vi "Finish.vi"   [LabVIEW 2012]
doc: "This VI is called just before exiting. It is expected to close I/O refnum, save collected data, etc."
uses:
  <vilib>/Rock Robotics/WPI/Compressor/WPI_CompressorGetSetRefNum.vi
  <vilib>/Rock Robotics/WPI/Joystick/WPI_JoystickGetSetRefNum.vi
  <vilib>/Rock Robotics/WPI/RobotDrive/WPI_RobotDriveGetSetRefNum.vi
types:
  T1 = typedef "WPI_EncoderDevRef.ctl" = cluster{"DevStatus":errorcluster, "EncoderIndex":T2, "CounterIndex":T3, "DistancePerCount":dbl, "Decoding Type":T4}
  T2 = typedef "FPGA_EncoderIdx.ctl" = enum8{"Enc 0", "Enc 1", "Enc 2", "Enc 3", "Invalid"}
  T3 = typedef "FPGA_CounterCtrSystemIndex.ctl" = enum8{"Ctr 0", "Ctr 1", "Ctr 2", "Ctr 3", "Ctr 4", "Ctr 5", "Ctr 6", "Ctr 7", "Invalid"}
  T4 = typedef "WPI_EncoderType.ctl" = enum16{"1x", "2x", "4x"}
  T5 = typedef "WPI_CompressorDevRef.ctl" = cluster{"DevStatus":errorcluster, "DigitalInputDevRef":T6, "RelayDevRef":T9}
  T6 = typedef "WPI_DigitalInputDevRef.ctl" = cluster{"DevStatus":errorcluster, "DIO Channel":T7, "Digital Module":T8}
  T7 = typedef "FPGA_DIOChannel.ctl" = enum8{"DIO 1", "DIO 2", "DIO 3", "DIO 4", "DIO 5", "DIO 6", "DIO 7", "DIO 8", "DIO 9", "DIO 10", "DIO 11", "DIO 12", "DIO 13", "DIO 14", "Invalid"}
  T8 = typedef "FPGA_TypedefDigitalModule.ctl" = enum16{"Digital Module 1", "Digital Module 2"}
  T9 = typedef "WPI_RelayDevRef.ctl" = cluster{"DevStatus":errorcluster, "Relay Channel":T10, "Digital Module":T8, "Relay Direction":T11}
  T10 = typedef "FPGA_DIORelayChannel.ctl" = enum8{"Relay 1", "Relay 2", "Relay 3", "Relay 4", "Relay 5", "Relay 6", "Relay 7", "Relay 8", "Invalid"}
  T11 = typedef "WPI_RelayDirection.ctl" = enum16{"Both directions", "Forward only", "Reverse only"}
  T12 = typedef "WPI_SolenoidDevRef.ctl" = cluster{"DevStatus":errorcluster, "Solenoid Module":T13, "Forward Solenoid Channel":T14, "Reverse Solenoid Channel":T14}
  T13 = typedef "FPGA_TypedefSolenoidModule.ctl" = enum16{"Solenoid Module 1", "Solenoid Module 2"}
  T14 = typedef "WPI_SolenoidChannel.ctl" = enum8{"Solenoid 1", "Solenoid 2", "Solenoid 3", "Solenoid 4", "Solenoid 5", "Solenoid 6", "Solenoid 7", "Solenoid 8", "Invalid"}
  T15 = typedef "WPI_CameraDevRef.ctl" = cluster{"Camera Address":string, "CameraStatus":errorcluster, "Acquire Image Notifier":refnum<notifier>}
  T16 = typedef "WPI_JoystickDevRef.ctl" = cluster{"Device":T17}
  T17 = typedef "WPI_JoystickDeviceEnum.ctl" = enum16{"USB 1", "USB 2", "USB 3", "USB 4", "Kinect 1", "Kinect 2"}
  T18 = typedef "WPI_RobotDriveDevRef.ctl" = cluster{"DevStatus":errorcluster, "Motors[]":T19[], "Square Inputs":bool, "Max Output":dbl, "Isochronous":bool}
  T19 = typedef "WPI_MotorControlDeviceRef.ctl" = cluster{"DeviceStatus":errorcluster, "Type":enum16{"PWM", "CAN"}, "PWM":cluster{"Digital Module":T8, "PWM Channel":T20, "DeadBand":T21}, "CAN":cluster{"Device Number":u8, "Control Mode":T22, "Semaphore":T23, "Max Vout":dbl}, "Invert":bool, "TransformRef":T24, "InvTransformRef":T24}
  T20 = typedef "FPGA_DIOPWMChannel.ctl" = enum8{"PWM 1", "PWM 2", "PWM 3", "PWM 4", "PWM 5", "PWM 6", "PWM 7", "PWM 8", "PWM 9", "PWM 10", "Invalid"}
  T21 = typedef "WPI_PWMDeadband.ctl" = cluster{"Name":string, "maxPositivePwm":i32, "minPositivePwm":i32, "centerPwm":i32, "maxNegativePwm":i32, "minNegativePwm":i32, "angularRange":u16}
  T22 = typedef "WPI_CANJaguar_ControlMode.ctl" = enum8{"Percent VBus", "Current", "Speed", "Position", "Voltage"}
  T23 = typedef "Semaphore RefNum" = refnum<k1>
  T24 = typedef "WPI_PWMTransform_ConPane.ctl" = refnum<vi>
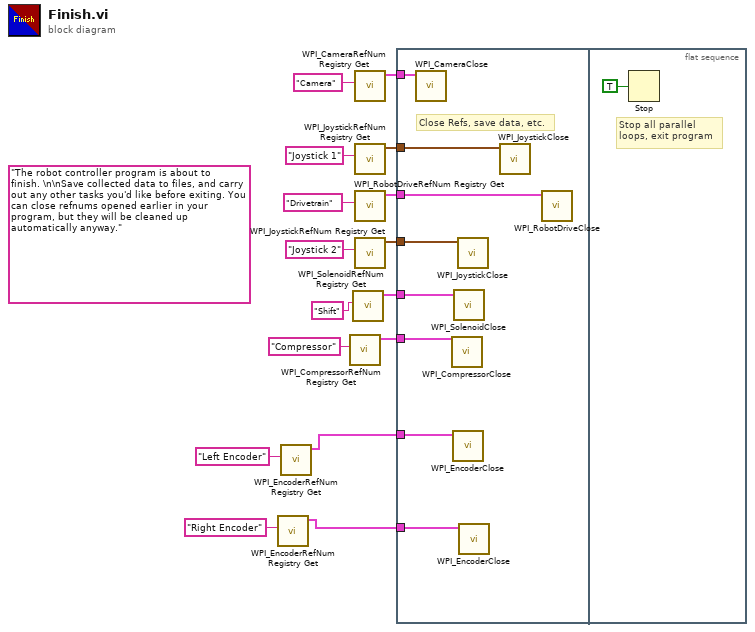
[diagram p0: block diagram]
diagram:
  (unwired) "The robot controller program is about to finish. \n\nSave collected data to files, and carry out any other tasks you'd like before exiting. You can close refnums opened earlier in your program, but they will be cleaned up automatically anyway."
  n1 = call <vilib>:"WPI_EncoderRefNum Registry Get.vi"("refnum name"="Right Encoder") -> ("EncoderDevRef"=w1:T1)  [unwired: 9 in, 1 out]
  n2 = call <vilib>:"WPI_EncoderRefNum Registry Get.vi"("refnum name"="Left Encoder") -> ("EncoderDevRef"=w2:T1)  [unwired: 9 in, 1 out]
  n3 = call <vilib>:"WPI_CompressorRefNum Registry Get.vi"("refnum name"="Compressor") -> ("CompressorDevRef"=w6:T5)  [unwired: 9 in, 1 out]
  n4 = call <vilib>:"WPI_SolenoidRefNum Registry Get.vi"("refnum name"="Shift") -> ("SolenoidDevRef"=w8:T12)  [unwired: 9 in, 1 out]
  n5 = call <vilib>:"WPI_CameraRefNum Registry Get.vi"("refnum name"="Camera") -> ("CameraDevRef"=w12:T15)  [unwired: 1 in, 9 out]
  n6 = call <vilib>:"WPI_JoystickRefNum Registry Get.vi"("refnum name"="Joystick 1") -> ("JoystickDevRef"=w13:T16)  [unwired: 1 in, 9 out]
  n7 = call <vilib>:"WPI_RobotDriveRefNum Registry Get.vi"("refnum name"="Drivetrain") -> ("RobotDriveDevRef"=w14:T18)  [unwired: 1 in, 9 out]
  n8 = call <vilib>:"WPI_JoystickRefNum Registry Get.vi"("refnum name"="Joystick 2") -> ("JoystickDevRef"=w9:T16)  [unwired: 1 in, 9 out]
  n9 = flat-sequence {
    tunnel: w14 -> [w24]
    tunnel: w13 -> [w23]
    tunnel: w12 -> [w22]
    tunnel: w9 -> [w21]
    tunnel: w8 -> [w20]
    tunnel: w6 -> [w19]
    tunnel: w2 -> [w18]
    tunnel: w1 -> [w17]
    frame #0 {
      # "Close Refs, save data, etc."
      n10 = call <vilib>:"WPI_CameraClose.vi"("CameraDevRef"=w22) -> ()  [unwired: 1 in, 10 out]
      n11 = call <vilib>:"WPI_CompressorClose.vi"("CompressorDevRef"=w19) -> ()  [unwired: 10 in, 1 out]
      n12 = call <vilib>:"WPI_EncoderClose.vi"("EncoderDevRef"=w18) -> ()  [unwired: 10 in, 1 out]
      n13 = call <vilib>:"WPI_SolenoidClose.vi"("SolenoidDevRef"=w20) -> ()  [unwired: 10 in, 1 out]
      n14 = call <vilib>:"WPI_JoystickClose.vi"("JoystickDevRef"=w21) -> ()  [unwired: 11 in]
      n15 = call <vilib>:"WPI_EncoderClose.vi"("EncoderDevRef"=w17) -> ()  [unwired: 10 in, 1 out]
      n16 = call <vilib>:"WPI_JoystickClose.vi"("JoystickDevRef"=w23) -> ()  [unwired: 11 out]
      n17 = call <vilib>:"WPI_RobotDriveClose.vi"("RobotDriveDevRef"=w24) -> ()  [unwired: 1 in, 10 out]
    }
    frame #1 {
      # "Stop all parallel\nloops, exit program"
      n18 = Stop(stop? (T)=TRUE ("Quit")) -> ()
    }
  }
